vi "RPI2 Enable UART.vi"(8 "Error In":errorcluster, 11 "Install LV Data":T1={"SSH Session"=refnum, "Status Log"="", "Detailed Log"="", "Credentials"={"Hostname or IP"="192.168.7.2", "Username"="root", "Password"=""}, "Target Info"={"OS Version"="", "CPU"="", "Systemd Version"="", "Internet Access"=FALSE, "Device Type"="", "LV Installed Ver"="", "LV Available Ver"="", "LV Upgrade Available"=FALSE, "Hostname"="", "NIC Info"=[]}, "Reboot Required?"=FALSE}) -> (0 "Error Out":errorcluster, 2 "Fixed?":bool, 3 "Install LV Data":T1={"SSH Session"=refnum, "Status Log"="", "Detailed Log"="", "Credentials"={"Hostname or IP"="192.168.7.2", "Username"="root", "Password"=""}, "Target Info"={"OS Version"="", "CPU"="", "Systemd Version"="", "Internet Access"=FALSE, "Device Type"="", "LV Installed Ver"="", "LV Available Ver"="", "LV Upgrade Available"=FALSE, "Hostname"="", "NIC Info"=[]}, "Reboot Required?"=FALSE})   [LabVIEW 2019, in "LMH-LINX.lvlib"]
uses:
  <vilib>/MakerHub/LINX/LMH-LINX.lvlib
  <vilib>/MakerHub/LINX/Private/Utilties/Target Management/Install LV Data.ctl
  E:/lv2019/dist/vi.lib/MakerHub/LINX/Resources/Renci.SshNet.dll
  Resources/Renci.SshNet.dll
  <vilib>/MakerHub/LINX/Private/Utilties/Target Management/Target Info.ctl
  <vilib>/MakerHub/LINX/Private/Utilties/Target Management/NIC Info.ctl
  <vilib>/MakerHub/LINX/Private/Utilties/Target Management/NIC Mode.ctl
  <vilib>/MakerHub/LINX/Private/Utilties/Target Management/Status FGV States.ctl
  <vilib>/regexp/Match Regular Expression.xnode
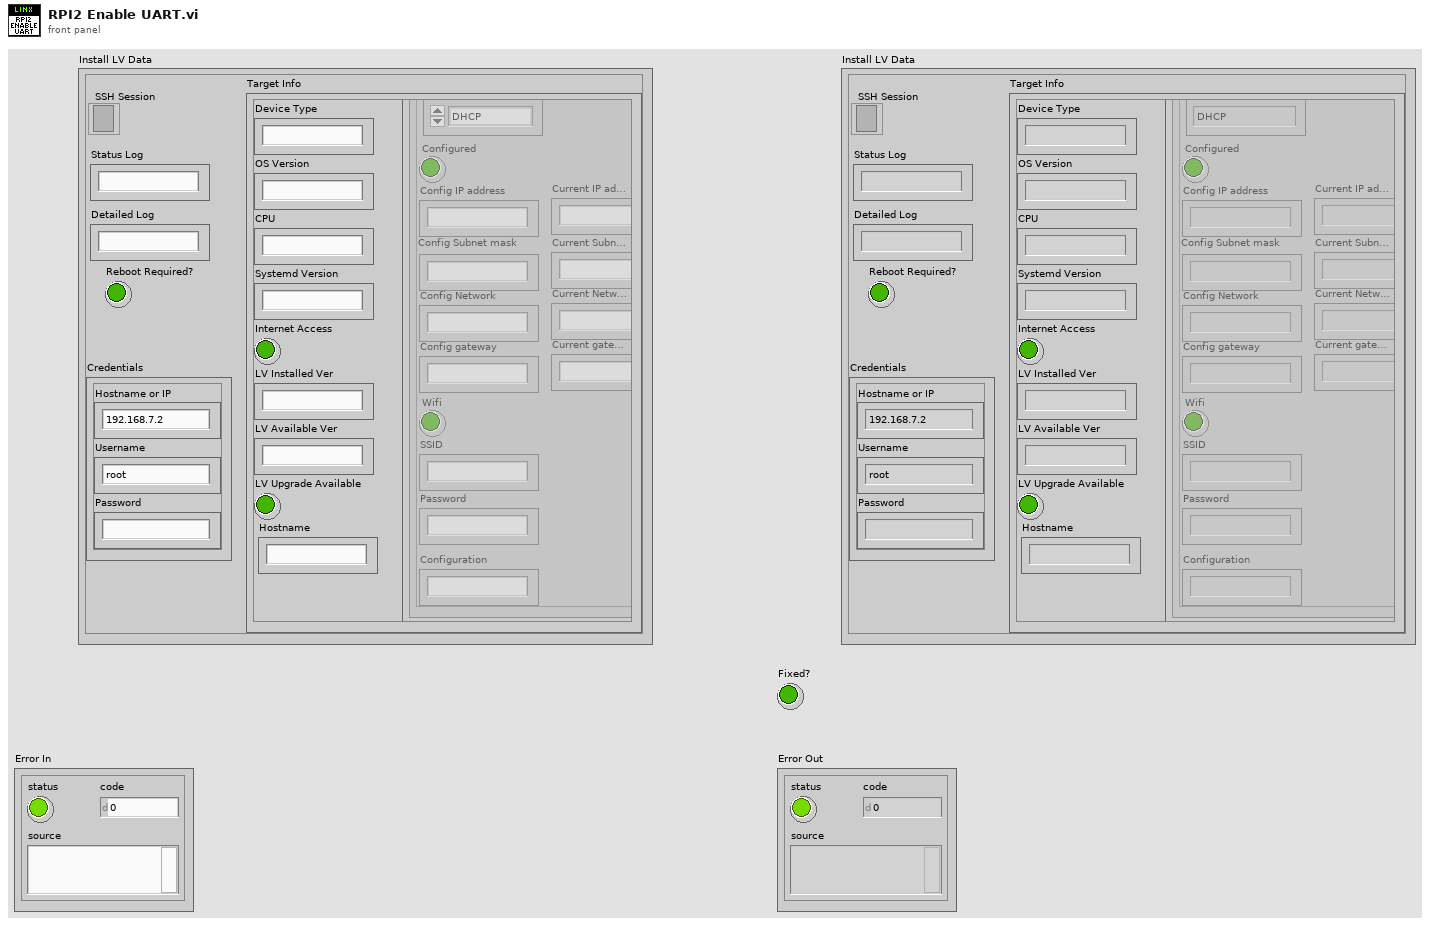
[diagram p1: front panel]
types:
  T1 = typedef "LMH-LINX.lvlib/Install LV Data.ctl" = cluster{"SSH Session":refnum<k24>, "Status Log":string, "Detailed Log":string, "Credentials":cluster{"Hostname or IP":string, "Username":string, "Password":string}, "Target Info":T2, "Reboot Required?":bool}
  T2 = typedef "LMH-LINX.lvlib/Target Info.ctl" = cluster{"OS Version":string, "CPU":string, "Systemd Version":string, "Internet Access":bool, "Device Type":string, "LV Installed Ver":string, "LV Available Ver":string, "LV Upgrade Available":bool, "Hostname":string, "NIC Info":T3[]}
  T3 = typedef "LMH-LINX.lvlib/NIC Info.ctl" = cluster{"Name":string, "NIC Mode":T4, "Configured":bool, "Config IP address":string, "Config Subnet mask":string, "Config Network":string, "Config gateway":string, "Wifi":bool, "SSID":string, "Password":string, "Configuration":string, "Current IP address":string, "Current Subnet mask":string, "Current gateway":string, "Current Network":string}
  T4 = typedef "LMH-LINX.lvlib/NIC Mode.ctl" = enum16{"DHCP", "Static", "Loopback"}
  T5 = typedef "LMH-LINX.lvlib/Status FGV States.ctl" = enum16{"Init", "Append", "Append History Only", "Set", "Get"}
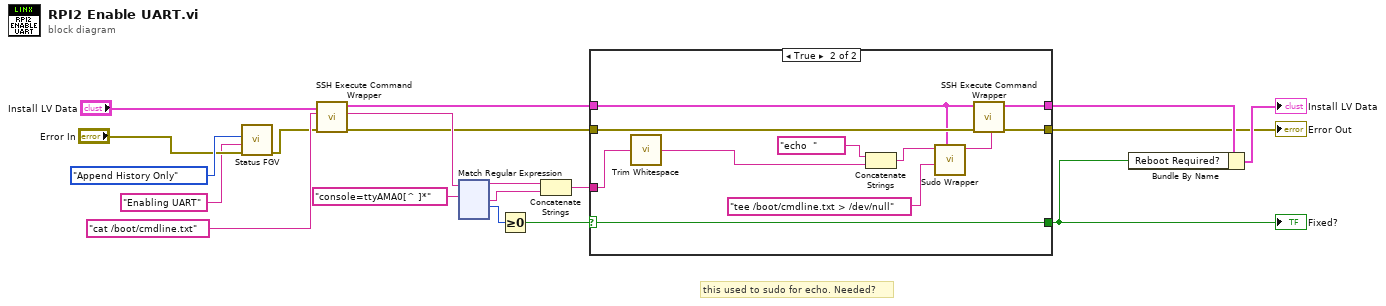
[diagram p0: block diagram]
diagram:
  # "this used to sudo for echo. Needed?"
  n1 = call <vilib>:"Status FGV.vi"("Error In"="Error In", "Status"="Enabling UART", "Status FGV State"=Status_FGV_States."Append History Only") -> ("Error Out"=w13:errorcluster)  [unwired: 6 in, 2 out]
  n2 = call <vilib>:"SSH Execute Command Wrapper.vi"("Error In"=w13, "Command"="cat /boot/cmdline.txt", "Install LV Data in"="Install LV Data") -> ("Error Out"=w9:errorcluster, "Std Out"=w14:string, "Install LV Data out"=w10:T1)  [unwired: 6 in]
  n3 = xnode "Match Regular Expression"("input string"=w14, "regular expression"="console=ttyAMA0[^ ]*" ("search string/char (-)")) -> ("before match"=w8:string, "after match"=w7:string, "offset past match"=w11:i32)  [unwired: 4 in, 2 out]
  n4 = Greater Or Equal To 0?(x=w11) -> (x >= 0?=w6:bool)
  n5 = Concatenate Strings(w8, w7) -> (w5:string)
  n6 = case shown="True" w6 {
    selector: w6 -> [w21 w32]
    tunnel: w10 -> [w22 w23]
    tunnel: w9 -> [w20 w29]
    tunnel: w5 -> [_ w28]
    tunnel: [w21 w32] -> w1
    tunnel: [w22 w31] -> w4
    tunnel: [w20 w30] -> w2
    frame False {
    }
    frame True {
      n7 = call <vilib>:"Trim Whitespace.vi"("string"=w28) -> ("trimmed string"=w27:string)  [unwired: 1 in]
      n8 = Concatenate Strings("echo  ", w27) -> (w25:string)
      n9 = call <vilib>:"Sudo Wrapper.vi"("Install LV Data"=w23, "comand string"="tee /boot/cmdline.txt > /dev/null" ("string"), "echo string"=w25) -> ("combined command string"=w26:string)  [unwired: 8 in]
      n10 = call <vilib>:"SSH Execute Command Wrapper.vi"("Error In"=w29, "Command"=w26, "Install LV Data in"=w23) -> ("Error Out"=w30:errorcluster, "Install LV Data out"=w31:T1)  [unwired: 6 in, 1 out]
    }
  }
  "Error Out" <- w2
  "Fixed?" <- w1
  n11 = Bundle By Name(cluster=w4, "Reboot Required?"=w1) -> (→"Install LV Data":T1)
